vi "Read QueueMessageRef.vi"(8 "error in (no error)":errorcluster, 11 "MicronGRPC in":refnum<class "MicronGRPC.lvclass">) -> (0 "error out":errorcluster, 2 "QueueMessageRef":refnum<queue>, 3 "MicronGRPC out":refnum<class "MicronGRPC.lvclass">)   [LabVIEW 2019, in "MicronGRPCGeneratedServer.lvlib" / "MicronGRPC.lvclass"]
uses:
  MicronGRPC.lvclass
  Base/Server/Message/MessageBase.lvclass
  MicronGRPC.lvclass/MicronGRPC.ctl
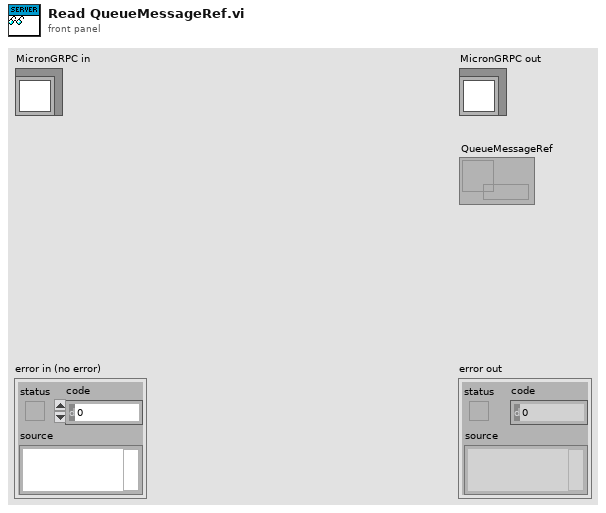
[diagram p1: front panel]
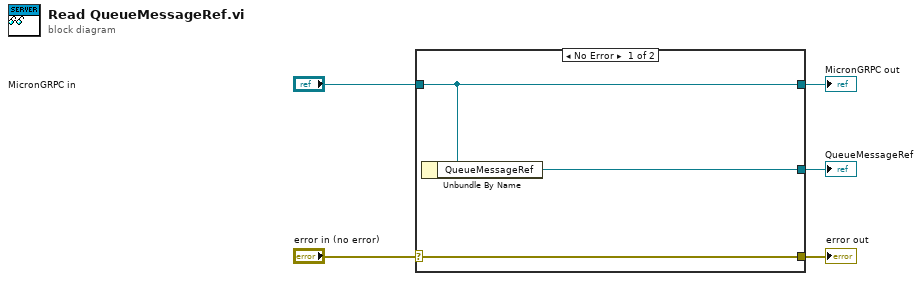
[diagram p0: block diagram]
diagram:
  n1 = case shown="No Error" "error in (no error)" {
    selector: "error in (no error)" -> [w8 w9]
    tunnel: [w8 w9] -> w4
    tunnel: [w7 w10] -> w2
    tunnel: "MicronGRPC in" -> [w7 w10]
    tunnel: [w6 _] -> w1
    frame No Error {
      n2 = Unbundle By Name(w7) -> ("QueueMessageRef"=w6:refnum<queue>)
    }
    frame Error {
    }
  }
  "error out" <- w4
  "MicronGRPC out" <- w2
  "QueueMessageRef" <- w1
